vi "xy file plot.vi"() -> ()   [LabVIEW 2021]
uses:
  <vilib>/Utility/file.llb/Read From Spreadsheet File (DBL).vi
panel:
  in  "Read":bool
  in  "#ofPins":i8
  in  "Continue":bool
  out "Data Array":dbl[][](array[numeric]) format="%.2f"
  out "X-Axis Array":dbl[][](array[numeric]) format="%.2f"
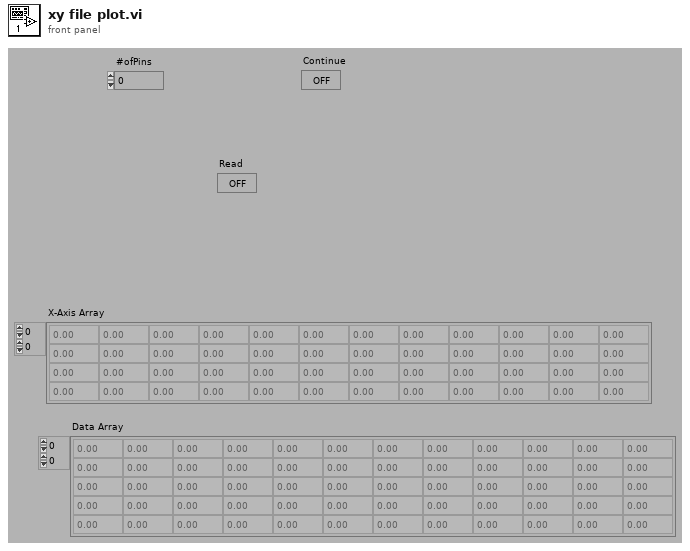
[diagram p1: front panel]
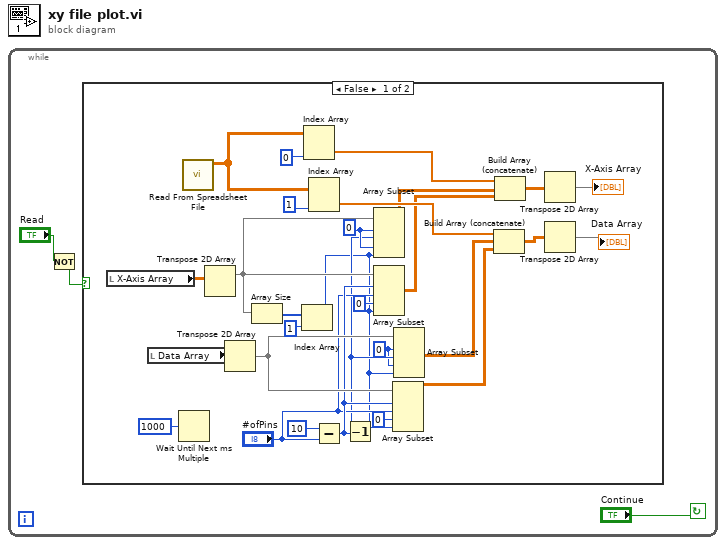
[diagram p0: block diagram]
diagram:
  n1 = while {
    stop <- "Continue" continue-if-true
    n2 = Not(x="Read") -> (.not. x?=w2:bool)
    n3 = case shown="False" w2 {
      frame False {
        w6 = 0
        w9 = 0
        n4 = local read "X-Axis Array"() -> (w19:dbl[][])
        n5 = local read "Data Array"() -> (w18:dbl[][])
        n6 = Wait Until Next ms Multiple(millisecond multiple=u32 1000) -> ()  [unwired: 1 out]
        n7 = call-poly <vilib>:"Read From Spreadsheet File.vi"() -> ("all rows"=w28:dbl[][])  [unwired: 7 in, 4 out]
        n8 = Transpose 2D Array(2D array=w19) -> (transposed array=w15:dbl[][])
        n9 = Transpose 2D Array(2D array=w18) -> (transposed array=w13:dbl[][])
        n10 = Array Size(array=w15) -> (size(s)=w22:i32[])
        n11 = Index Array(array=w22, index=1) -> (element=w5:i32)
        n12 = Index Array(array=w28, index (col)=0) -> (element=w32:dbl[])  [unwired: 1 in]
        n13 = Index Array(array=w28, index (col)=1) -> (element=w31:dbl[])  [unwired: 1 in]
        n14 = Subtract(x=10, y="#ofPins") -> (x-y=w11:i32)
        n15 = Decrement(x=w11) -> (x-1=w7:i32)
        n16 = Array Subset(array=w15, index (row)=w9, length (row)=w7, index (col)=w9, length (col)=w5) -> (w21:dbl[][])
        n17 = Array Subset(array=w15, index (row)=w11, length (row)="#ofPins", index (col)=0, length (col)=w5) -> (w14:dbl[][])
        n18 = Array Subset(array=w13, index (row)=w11, length (row)="#ofPins", index (col)=0, length (col)=w5) -> (w12:dbl[][])
        n19 = Array Subset(array=w13, index (row)=w6, length (row)=w7, index (col)=w6, length (col)=w5) -> (w20:dbl[][])
        n20 = Build Array (concatenate)(w31, w20, w12) -> (w26:dbl[][])
        n21 = Build Array (concatenate)(w32, w21, w14) -> (w27:dbl[][])
        n22 = Transpose 2D Array(2D array=w27) -> (transposed array=→"X-Axis Array":dbl[][])
        n23 = Transpose 2D Array(2D array=w26) -> (transposed array=→"Data Array":dbl[][])
      }
      frame True {
      }
    }
  }
